vi "Launcher - Test Timer.vi"(6 "Worker Alias":string="Test Timer", 9 "Initialization Data":T1, 11 "Test Timer in":refnum<class "Test Timer.lvclass">) -> (0 "error out":errorcluster)   [LabVIEW 2021]
doc: "This VI launches the Head Worker of a Workers application."
uses:
  Workers/Test Timer/Test Timer.lvclass
  <vilib>/addons/_Workers/Debugger/Debug Client/Debug Client.lvlib
  Workers/Test Timer/Response Cases.ctl
  Workers/Test Timer/Initialization Data.ctl
panel:
  # "Launches the Timer Worker test program\n\nThe Timer worker provides the same functionality as the Actor frameworks Time Delayed Send Message.vi"
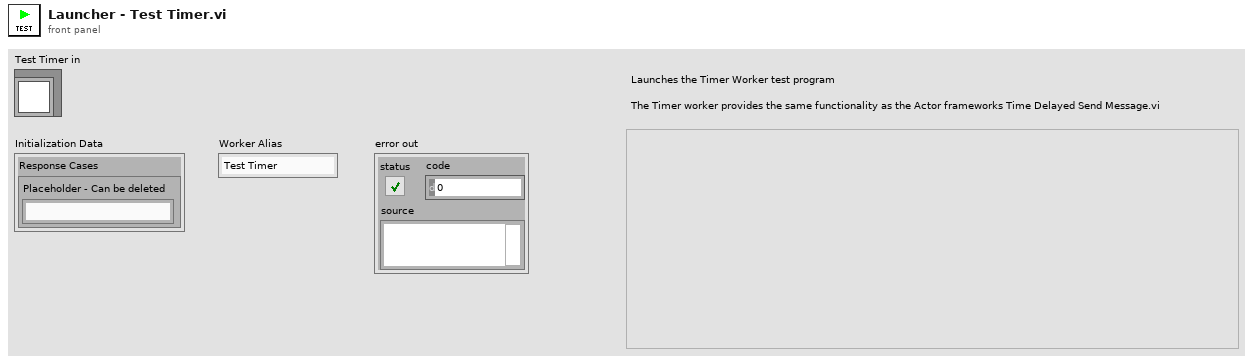
[diagram p1: front panel]
types:
  T1 = typedef "Test Timer.lvclass/Initialization Data.ctl" = cluster{"Response Cases":T2}
  T2 = typedef "Test Timer.lvclass/Response Cases.ctl" = cluster{"Placeholder - Can be deleted":string}
  T3 = enum32{"Invalid", "Standard", "Closed", "Hidden", "Minimized", "Maximized"}
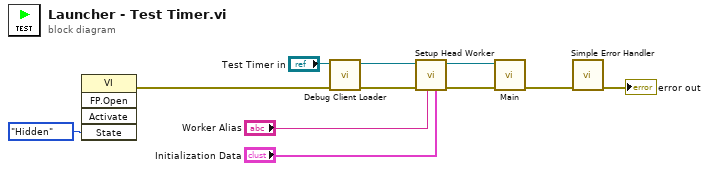
[diagram p0: block diagram]
diagram:
  n1 = invoke class="VI" method="FP.Open"("State"=T3."Hidden") -> (error out=w1:errorcluster)  [unwired: 4 in, 4 out]
  n2 = call <vilib>:"Debug Client Loader.vi"("error in (no error)"=w1, "Worker_"="Test Timer in") -> ("error out"=w5:errorcluster, "Worker_out"=w4:refnum<class "Test Timer.lvclass">)  [unwired: 8 in]
  n3 = call-dynamic "Setup Head Worker.vi"("Initalization Data"="Initialization Data", "Worker Alias"="Worker Alias", "error in"=w5, "Worker_"=w4) -> ("error out"=w11:errorcluster, "Worker_out"=w9:refnum<class "Test Timer.lvclass">)  [unwired: 6 in]
  n4 = call-dynamic "Main.vi"("error in"=w11, "Test Timer in"=w9) -> ("error out"=w10:errorcluster)  [unwired: 8 in, 1 out]
  n5 = call <vilib>:"Simple Error Handler.vi"("error in (no error)"=w10) -> ("error out"=→"error out":errorcluster)  [unwired: 4 in, 4 out]
